vi "ECOG Monitor.vi"() -> ()   [LabVIEW 2020]
uses:
  Typedefs/ECOG-State.ctl
  Typedefs/ECOG-Parameters.ctl
  <vilib>/DAQmx/read.llb/DAQmx Read (Analog 1D DBL 1Chan NSamp).vi
  <extravilib>/ChannelInstances/Stream-a[.](dbl)/Read With Abort.vi
  <extravilib>/ChannelInstances/Stream-a[.](dbl)/Write With Abort.vi
  <extravilib>/ChannelInstances/Stream-a[.](dbl)/EndpointRead.vi
  <extravilib>/ChannelInstances/Stream-a[.](dbl)/Endpoint.vi
  <extravilib>/ChannelInstances/Stream-a[.](dbl)/Instantiate.vi
  <extravilib>/ChannelInstances/Stream-a[.](dbl)/)Channel.vi
  <resource>/ChannelSupport/_ChannelSupport/WaitIfNeeded.vi
  <vilib>/DAQmx/miscellaneous.llb/DAQmx Fill In Error Info.vi
  <extravilib>/ChannelInstances/Stream-a[.](dbl).lvlib
panel:
  in  "Filter":bool
  in  "Start":bool
  in  "Stop":bool
  out "Graph":cluster{dbl[], dbl[]}(graph)
  in  "result":T1
  out "Map":dbl[][](graph)
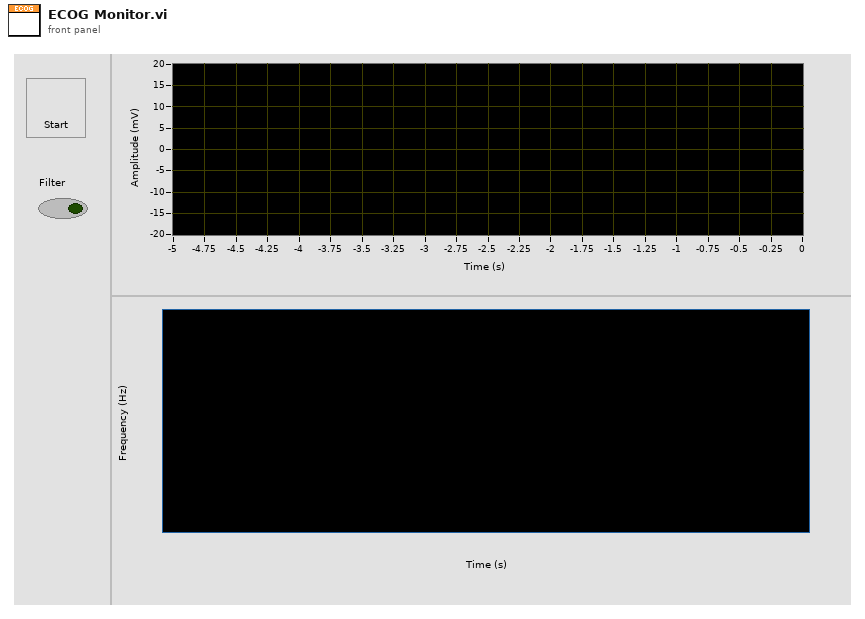
[diagram p1: front panel]
types:
  T1 = cluster{"status":string, "finished":errorcluster}
  T2 = typedef "ECOG-Parameters.ctl" = cluster{"Channel":string, "Fs":dbl, "Frame Size":dbl, "History Length":dbl, "Filter":bool, "Flo":dbl, "Fhi":dbl, "Fmax":dbl, "Splitter Position":i32}
  T3 = typedef "ECOG-State.ctl" = cluster{"running":bool}
  T4 = enum8{"Enabled", "Disabled", "Disabled and Grayed Out"}
  T5 = cluster{string, "\"Settings\" or \"Parameters\"":T2}
  T6 = typedef "ECOG-Spectrogram.ctl" = cluster{"ref":refnum<vi>, "nacq":i32, "map":dbl[][], "nmax":i32}
  T7 = typedef "ECOG-Display.ctl" = cluster{"ref":refnum<vi>, "chart":cluster{"time":dbl[], "y":dbl[]}, "nacq":i32, "nmax":i32, "IIR Filter":cluster{"filter structure":enum32{"IIR 2nd Order", "IIR 4th Order"}, "Reverse Coefficients":dbl[], "Forward Coefficients":dbl[]}, "Final Filter State":dbl[]}
  T8 = typedef "Stream-a[.](dbl).lvlib/)Channel.ctl" = refnum<queue>
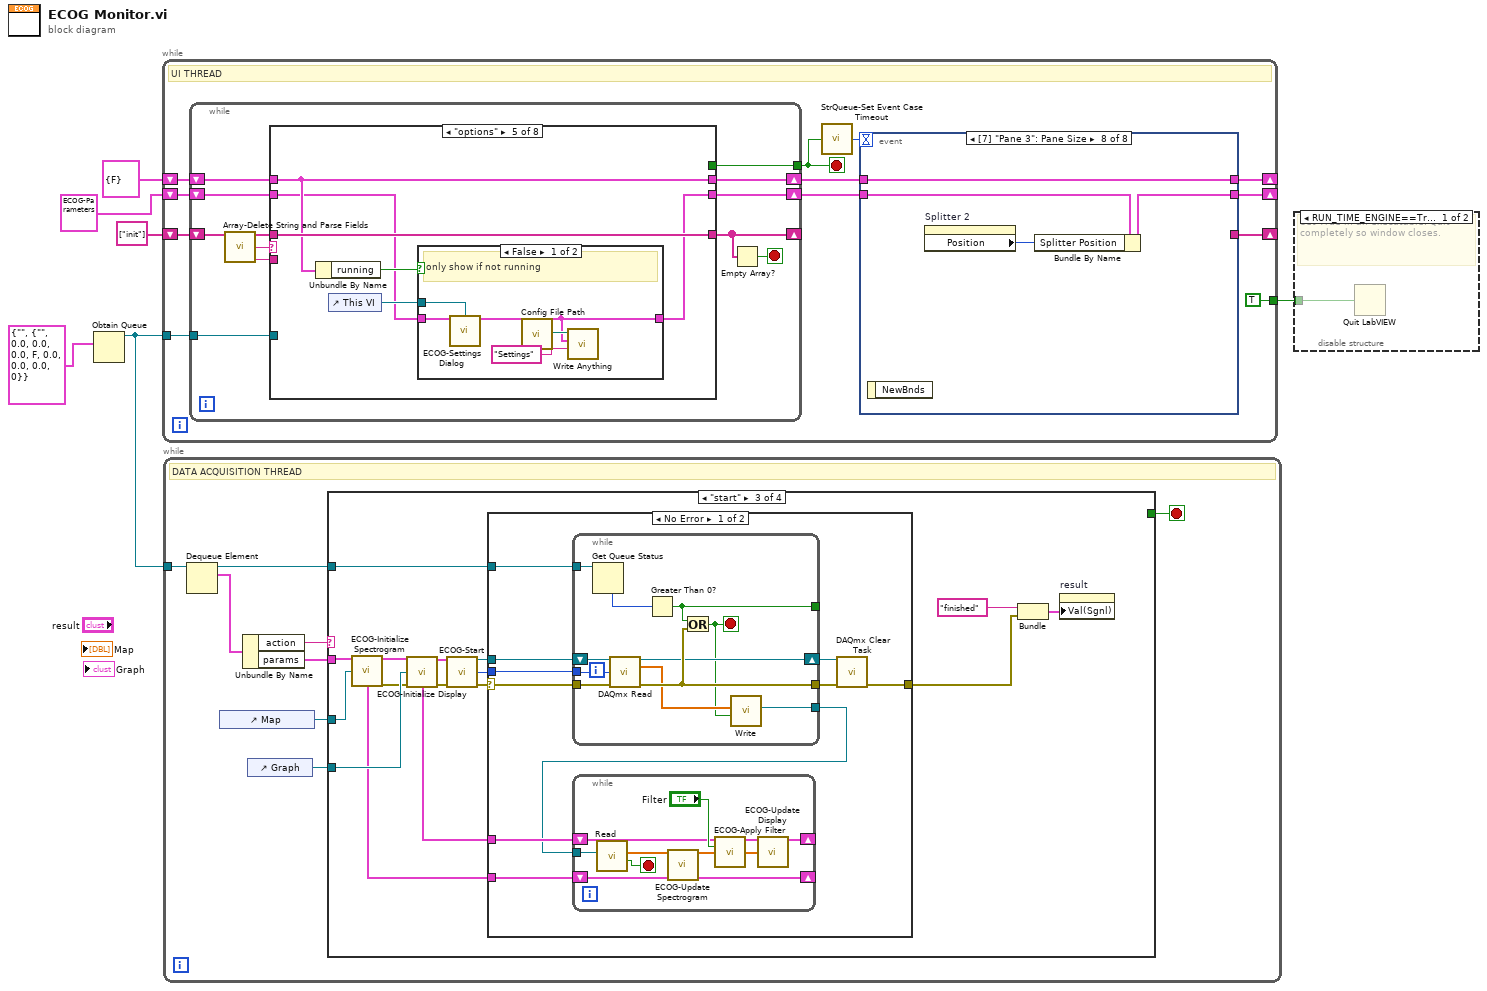
[diagram p0: block diagram]
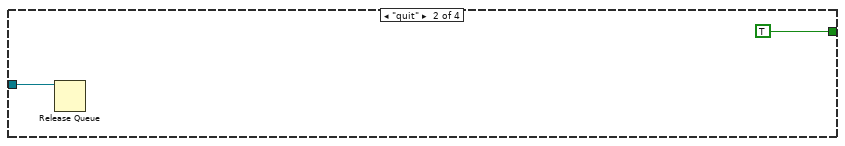
[diagram p3: hidden frame]
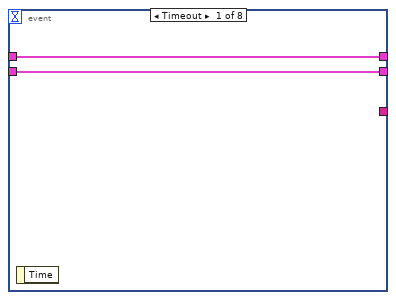
[diagram p6: hidden frame]
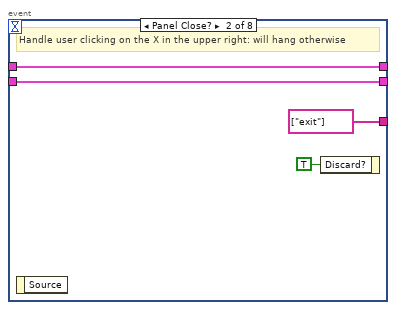
[diagram p7: hidden frame]
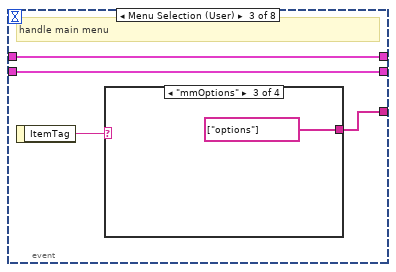
[diagram p8: hidden frame]
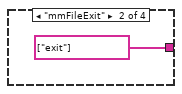
[diagram p10: hidden frame]
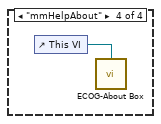
[diagram p11: hidden frame]
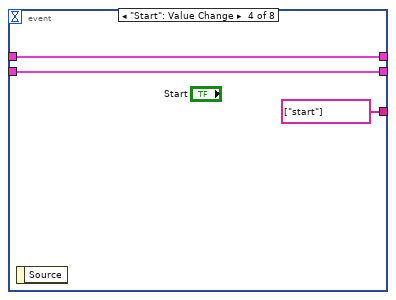
[diagram p12: hidden frame]
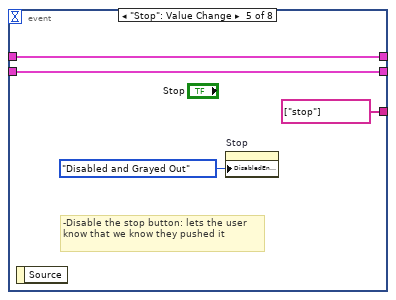
[diagram p13: hidden frame]
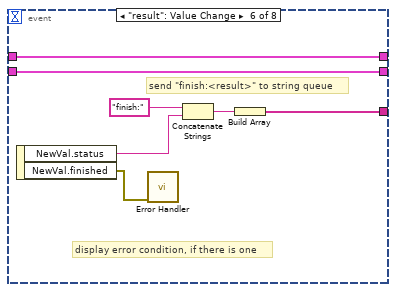
[diagram p14: hidden frame]
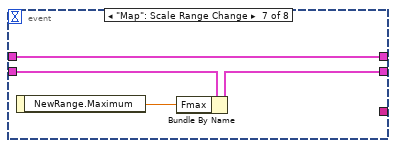
[diagram p15: hidden frame]
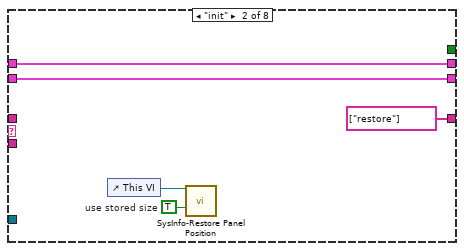
[diagram p17: hidden frame]
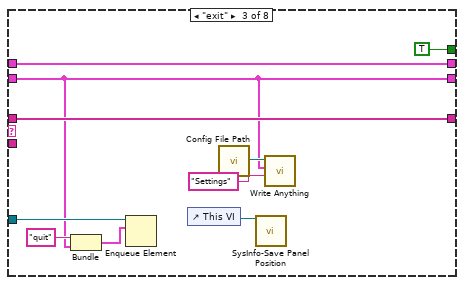
[diagram p18: hidden frame]
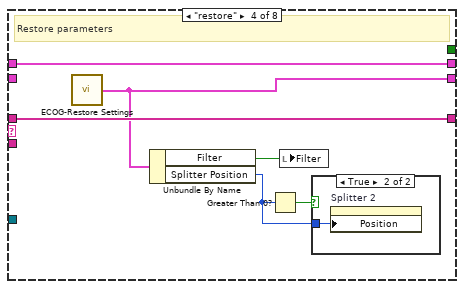
[diagram p19: hidden frame]
diagram:
  n1 = Obtain Queue(element data type=cluster{"action":string, "params":T2} {"action"="", "params"={"Channel"="", "Fs"=0.0, "Frame Size"=0.0, "History Length"=0.0, "Filter"=FALSE, "Flo"=0.0, "Fhi"=0.0, "Fmax"=0.0, "Splitter Position"=0}}) -> (queue out=w2:refnum<queue>)  [unwired: 4 in, 2 out]
  n2 = while {
    shift-right: [w15] -> _
    shift-left: string[] ["init"] -> [w16]
    shift-right: [w12] -> _
    shift-left: T3 {"running"=FALSE} ("State") -> [w14]
    shift-right: [w9] -> _
    shift-left: T2 {"Channel"="", "Fs"=0.0, "Frame Size"=0.0, "History Length"=0.0, "Filter"=FALSE, "Flo"=0.0, "Fhi"=0.0, "Fmax"=0.0, "Splitter Position"=0} ("\"Settings\" or \"Parameters\"") -> [w11]
    tunnel: [TRUE] -> w3
    tunnel: w2 -> [w7]
    stop <- w18 stop-if-true
    # "UI THREAD"
    n3 = while {
      shift-right: [w65] -> _
      shift-left: w16 -> [w62]
      tunnel: [w63] -> w18
      shift-right: [w58] -> w13
      shift-left: w14 -> [w59]
      shift-right: [w56] -> w10
      shift-left: w11 -> [w57]
      tunnel: w7 -> [w55]
      stop <- w64 stop-if-true
      n4 = call "Array-Delete String and Parse Fields.vi"("Array in"=w62) -> ("Array out"=w61:string[], "Field 1"=w60:string, "Field 2"=w54:string)  [unwired: 10 in, 2 out]
      n5 = case shown="\"options\"" w60 {
        tunnel: w61 -> [w68 _ w83 w89 w96 w112 w118 w124]
        tunnel: [w68 string[] ["restore"] ("Array out") w83 w89 w96 w112 w118 w124] -> w65
        tunnel: [_ _ TRUE _ _ _ _ _] -> w63
        tunnel: w59 -> [w67 w73 w81 w88 w93 w111 w117 w123]
        tunnel: [w67 w73 w81 w88 w93 w104 w117 w120] -> w58
        tunnel: w57 -> [w66 w72 w74 _ w92 w107 w113 w122]
        tunnel: [w66 w72 w74 w87 w91 w107 w113 w122] -> w56
        tunnel: w55 -> [_ _ w79 _ _ w108 w114 _]
        tunnel: w54 -> [_ _ _ _ _ _ _ _]
        frame "", Default {
        }
        frame "init" {
          w69 = TRUE  # use stored size
          n6 = control-ref of="This VI"() -> (w71:refnum<vi>)
          n7 = call "SysInfo-Restore Panel Position.vi"("VI Refnum"=w71, "use stored size"=w69) -> ()  [unwired: 11 in, 3 out]
        }
        frame "exit" {
          n8 = Bundle("quit", "\"Settings\" or \"Parameters\""=w74) -> (w77:T5)  [unwired: 1 in]
          n9 = Enqueue Element(queue=w79, element=w77) -> ()  [unwired: 2 in, 3 out]
          n10 = control-ref of="This VI"() -> (w80:refnum<vi>)
          n11 = call "Config File Path.vi"() -> ("Default config file name"=w75:path)  [unwired: 1 in]
          n12 = call "SysInfo-Save Panel Position.vi"("VI Refnum"=w80) -> ()  [unwired: 14 in, 1 out]
          n13 = call "Write Anything.vi"("Section Name (Name of \"Anything\")"="Settings" ("Section Name (Name of \"Type of Anything\")"), "Anything"=w74, "Path (dialog)"=w75) -> ()  [unwired: 7 in, 2 out]
        }
        frame "restore" {
          # "Restore parameters"
          n14 = call "ECOG-Restore Settings.vi"() -> ("Settings"=w87:T2)  [unwired: 15 in]
          n15 = Unbundle By Name(w87) -> ("Filter"=w86:bool, "Splitter Position"=w85:i32)
          n16 = Greater Than 0?(x=w85) -> (x > 0?=w84:bool)
          n17 = local write "Filter"(w86) -> ()
          n18 = case shown="True" w84 {
            tunnel: w85 -> [_ w90]
            frame False {
            }
            frame True {
              n19 = property on="Splitter 2" class="Splitter"("Position"=w90) -> ()  [unwired: 2 in, 2 out]
            }
          }
        }
        frame "options" {
          n20 = Unbundle By Name(w93) -> ("running"=w95:bool)
          n21 = control-ref of="This VI"() -> (w94:refnum<vi>)
          n22 = case shown="False" w95 {
            tunnel: w94 -> [w101 _]
            tunnel: w92 -> [w100 w102]
            tunnel: [w97 w102] -> w91
            frame False {
              # "only show if not running"
              n23 = call "ECOG-Settings Dialog.vi"("Settings in"=w100, "Parent VI"=w101) -> ("Settings out"=w97:T2)  [unwired: 12 in, 1 out]
              n24 = call "Config File Path.vi"() -> ("Default config file name"=w99:path)  [unwired: 1 in]
              n25 = call "Write Anything.vi"("Section Name (Name of \"Anything\")"="Settings" ("Section Name (Name of \"Type of Anything\")"), "Anything"=w97, "Path (dialog)"=w99) -> ()  [unwired: 7 in, 2 out]
            }
            frame True {
            }
          }
        }
        frame "start" {
          # "Make sure Stop is enabled"
          n26 = Bundle("start", "\"Settings\" or \"Parameters\""=w107) -> (w109:T5)  [unwired: 1 in]
          n27 = Enqueue Element(queue=w108, element=w109) -> ()  [unwired: 2 in, 3 out]
          n28 = property on="Stop" class="Bool"("DisabledEnum"=T4."Enabled" ("Disabled")) -> ()  [unwired: 2 in, 2 out]
          n29 = property on="Start" class="Bool"("Visible"=FALSE) -> ()  [unwired: 2 in, 2 out]
          n30 = Bundle By Name(cluster=w111, "running"=TRUE) -> (w104:T3)
        }
        frame "stop" {
          n31 = Bundle("stop", "\"Settings\" or \"Parameters\""=w113) -> (w115:T5)  [unwired: 1 in]
          n32 = Enqueue Element(queue=w114, element=w115) -> ()  [unwired: 2 in, 3 out]
        }
        frame "finish" {
          # "the instruction sent by the \"result\" Event case is in the form \"finish:<result>\""
          n33 = property on="Start" class="Bool"("Visible"=TRUE) -> ()  [unwired: 2 in, 2 out]
          n34 = Bundle By Name(cluster=w123, "running"=FALSE) -> (w120:T3)
        }
      }
      n35 = Empty Array?(array=w65) -> (empty?=w64:bool)
    }
    n36 = call "StrQueue-Set Event Case Timeout.vi"("Quit"=w18) -> ("timeout"=w17:i32)  [unwired: 14 in]
    n37 = event shown="[7] \"Pane 3\": Pane Size" {
      selector: _ -> [_ _ _ _ _ _ _ _]
      dyn-events: _ -> [_ _ _ _ _ _ _ _]
      timeout: w17 -> [_ _ _ _ _ _ _ _]
      tunnel: [_ string[] ["exit"] w25 string[] ["start"] string[] ["stop"] w39 _ _] -> w15
      tunnel: w13 -> [w20 w22 w28 w34 w38 w45 w49 w53]
      tunnel: [w20 w22 w28 w34 w38 w45 w49 w53] -> w12
      tunnel: w10 -> [w19 w21 w27 w33 w37 w44 w48 w52]
      tunnel: [w19 w21 w27 w33 w37 w44 w47 w51] -> w9
      event Timeout {
        n38 = event-data() -> ()  [unwired: 1 in, 1 out]
      }
      event Panel Close? {
        # "Handle user clicking on the X in the upper right: will hang otherwise"
        n39 = event-data() -> ()  [unwired: 1 in, 1 out]
        n40 = event-data("Discard?"=TRUE) -> ()  [unwired: 1 in, 1 out]
      }
      event Menu Selection (User) {
        # "handle main menu"
        n41 = event-data() -> ("ItemTag"=w26:string)  [unwired: 1 in]
        n42 = case shown="\"mmOptions\"" w26 {
          tunnel: [_ string[] ["exit"] string[] ["options"] _] -> w25
          frame "", Default {
          }
          frame "mmFileExit" {
          }
          frame "mmOptions" {
          }
          frame "mmHelpAbout" {
            n43 = control-ref of="This VI"() -> (w31:refnum<vi>)
            n44 = call "ECOG-About Box.vi"("Parent VI"=w31) -> ()  [unwired: 15 in]
          }
        }
      }
      event "Start": Value Change {
        n45 = event-data() -> ()  [unwired: 1 in, 1 out]
      }
      event "Stop": Value Change {
        # "-Disable the stop button: lets the user know that we know they pushed it"
        n46 = event-data() -> ()  [unwired: 1 in, 1 out]
        n47 = property on="Stop" class="Bool"("DisabledEnum"=T4."Disabled and Grayed Out" ("Disabled")) -> ()  [unwired: 2 in, 2 out]
      }
      event "result": Value Change {
        # "send \"finish:<result>\" to string queue"
        # "display error condition, if there is one"
        n48 = event-data() -> ("NewVal.status"=w42:string, "NewVal.finished"=w41:errorcluster)  [unwired: 1 in]
        n49 = call "Error Handler.vi"("error in (no error)"=w41) -> ()  [unwired: 12 in, 3 out]
        n50 = Concatenate Strings("finish:" ("string"), w42) -> (w40:string)
        n51 = Build Array(w40) -> (w39:string[])
      }
      event "Map": Scale Range Change {
        n52 = event-data() -> ("NewRange.Maximum"=w46:dbl)  [unwired: 1 in]
        n53 = Bundle By Name(cluster=w48, "Fmax"=w46) -> (w47:T2)
      }
      event Pane Size {
        n54 = event-data() -> ()  [unwired: 1 in, 1 out]
        n55 = property on="Splitter 2" class="Splitter"() -> ("Position"=w50:i32)  [unwired: 2 in, 2 out]
        n56 = Bundle By Name(cluster=w52, "Splitter Position"=w50) -> (w51:T2)
      }
    }
  }
  n57 = while {
    tunnel: w2 -> [w132]
    stop <- w129 stop-if-true
    # "DATA ACQUISITION THREAD"
    n58 = Dequeue Element(queue=w132) -> (queue out=w127:refnum<queue>, element=w128:cluster{"action":string, "params":T2})  [unwired: 2 in, 2 out]
    n59 = control-ref of="Map"() -> (w125:refnum<vi>)
    n60 = Unbundle By Name(w128) -> ("action"=w131:string, "params"=w130:T2)
    n61 = control-ref of="Graph"() -> (w126:refnum<vi>)
    n62 = case shown="\"start\"" w131 {
      tunnel: w130 -> [_ _ w139 _]
      tunnel: [_ TRUE _ _] -> w129
      tunnel: w127 -> [_ w133 w150 _]
      tunnel: w126 -> [_ _ w141 _]
      tunnel: w125 -> [_ _ w135 _]
      frame "", Default {
      }
      frame "quit" {
        n63 = Release Queue(queue=w133) -> ()  [unwired: 2 in, 3 out]
      }
      frame "start" {
        n64 = call "ECOG-Initialize Spectrogram.vi"("params"=w139, "Map Ref"=w135) -> ("params thru"=w138:T2, "spectrogram"=w136:T6, "error out"=w137:errorcluster)  [unwired: 11 in]
        n65 = call "ECOG-Initialize Display.vi"("params"=w138, "ref"=w141, "error in (no error)"=w137) -> ("params thru"=w143:T2, "display"=w140:T7, "error out"=w142:errorcluster)  [unwired: 10 in]
        n66 = call "ECOG-Start.vi"("params"=w143, "error in (no error)"=w142) -> ("task out"=w146:refnum<k21>, "nread"=w144:i32, "error out"=w147:errorcluster)  [unwired: 11 in]
        n67 = case shown="No Error" w147 {
          selector: w147 -> [w159 w183]
          tunnel: w150 -> [w160 _]
          tunnel: w146 -> [w158 _]
          tunnel: w144 -> [w157 _]
          tunnel: [w154 w183] -> w145
          tunnel: w140 -> [w153 _]
          tunnel: w136 -> [w151 _]
          frame No Error {
            n68 = while {
              tunnel: w160 -> [w182]
              tunnel: [w177] -> _
              tunnel: w159 -> [w179]
              tunnel: w157 -> [w178]
              tunnel: [w176] -> w155
              shift-right: [w175] -> w156
              shift-left: w158 -> [w180]
              tunnel: [w172] -> w152
              stop <- w173 stop-if-true
              n69 = Get Queue Status(queue=w182) -> (# elements in queue=w181:i32)  [unwired: 2 in, 7 out]
              n70 = call-poly <vilib>:"DAQmx Read.vi"("task/channels in"=w180, "number of samples per channel"=w178, "error in"=w179) -> ("task out"=w175:refnum<k21>, "data"=w174:dbl[], "error out"=w176:errorcluster)  [unwired: 10 in]
              n71 = Greater Than 0?(x=w181) -> (x > 0?=w177:bool)
              n72 = Or(x=w177, y=w176) -> (x .or. y?=w173:bool)
              n73 = call <extravilib>:"Write.vi"("last element? (F)"=w173, "element"=w174) -> ("channel"=w172:T8)  [unwired: 7 in, 2 out]
            }
            n74 = while {
              tunnel: w152 -> [w171]
              shift-right: [w169] -> _
              shift-left: w153 -> [w165]
              shift-right: [w161] -> _
              shift-left: w151 -> [w162]
              stop <- w170 stop-if-true
              n75 = call <extravilib>:"Read.vi"("channel"=w171) -> ("last element?"=w170:bool, "element"=w164:dbl[])  [unwired: 6 in, 3 out]
              n76 = call "ECOG-Update Spectrogram.vi"("new data"=w164, "spectrogram in"=w162) -> ("new data thru"=w163:dbl[], "spectrogram out"=w161:T6)  [unwired: 12 in]
              n77 = call "ECOG-Apply Filter.vi"("display in"=w165, "Filter?"="Filter", "new data"=w163) -> ("display out"=w167:T7, "Filtered X"=w168:dbl[])  [unwired: 11 in]
              n78 = call "ECOG-Update Display.vi"("display in"=w167, "new data"=w168) -> ("display out"=w169:T7)  [unwired: 13 in]
            }
            n79 = call <vilib>:"DAQmx Clear Task.vi"("task in"=w156, "error in"=w155) -> ("error out"=w154:errorcluster)  [unwired: 13 in]
          }
          frame Error {
          }
        }
        n80 = Bundle("finished", "error IO"=w145) -> (w148:cluster{string, "error IO":errorcluster})  [unwired: 1 in]
        n81 = property on="result" class="Clust (strict)"("Val(Sgnl)"=w148) -> ()  [unwired: 2 in, 2 out]
      }
      frame "stop" {
      }
    }
  }
  n82 = disable-structure shown="RUN_TIME_ENGINE==True" {
    disable-tunnel: w3 -> [w184 _]
    frame condition #0 {
      # "Set True in an executable. Quit completely so window closes."
      n83 = Quit LabVIEW(quit? (T)=w184) -> ()
    }
    frame condition #1 (active) {
      # "Running in LabVIEW development system. Leaves window open"
    }
  }
